vi "TCP_IP_N6705B_Press_Datalog_button.vi"(8 "error in (no error)":errorcluster, 11 "instrument address":string) -> (0 "error out":errorcluster)   [LabVIEW 2015]
panel:
  out "Numeric":i32
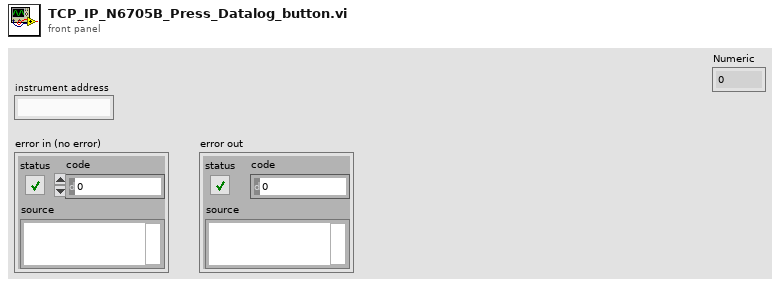
[diagram p1: front panel]
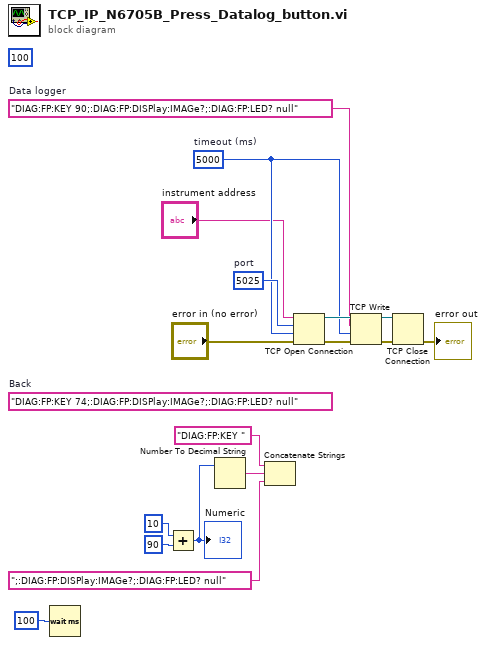
[diagram p0: block diagram]
diagram:
  (unwired) "DIAG:FP:KEY 74;:DIAG:FP:DISPlay:IMAGe?;:DIAG:FP:LED? null"  # Back
  w1 = "DIAG:FP:KEY 90;:DIAG:FP:DISPlay:IMAGe?;:DIAG:FP:LED? null"  # Data logger
  w14 = u16 5025  # port
  w11 = 5000  # timeout (ms)
  (unwired) 100
  n1 = Wait (ms)(milliseconds to wait=u32 100) -> ()  [unwired: 1 out]
  n2 = Add(x=10, y=90) -> (x+y=w4:i32)
  "Numeric" <- w4
  n3 = Number To Decimal String(number=w4) -> (decimal integer string=w6:string)  [unwired: 1 in]
  n4 = Concatenate Strings("DIAG:FP:KEY " ("string"), w6, ";:DIAG:FP:DISPlay:IMAGe?;:DIAG:FP:LED? null" ("string")) -> ()  [unwired: 1 out]
  n5 = TCP Open Connection(address="instrument address", remote port or service name=w14, timeout ms (60000)=w11, error in (no error)="error in (no error)") -> (connection ID=w15:refnum<k5>, error out=w16:errorcluster)  [unwired: 1 in]
  n6 = TCP Write(connection ID=w15, data in=w1, error in (no error)=w16, 9:w11) -> (connection ID out=w12:refnum<k5>, error out=w13:errorcluster)  [unwired: 1 out]
  n7 = TCP Close Connection(connection ID=w12, error in (no error)=w13) -> (error out=→"error out":errorcluster)  [unwired: 1 in, 1 out]
